vi "Write Version.vi"(8 "error in":errorcluster, 10 "Version":string, 11 "Custom Device Config in":refnum<class "Custom Device Config.lvclass">) -> (0 "error out":errorcluster, 3 "Custom Device Config out":refnum<class "Custom Device Config.lvclass">)   [LabVIEW 2024, in "Parser.lvlib" / "Custom Device Config.lvclass"]
uses:
  Custom Device Config.lvclass
  Custom Device Config.lvclass/Custom Device Config.ctl
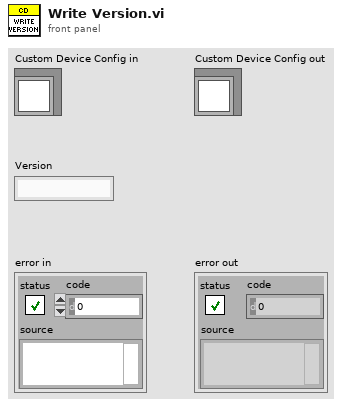
[diagram p1: front panel]
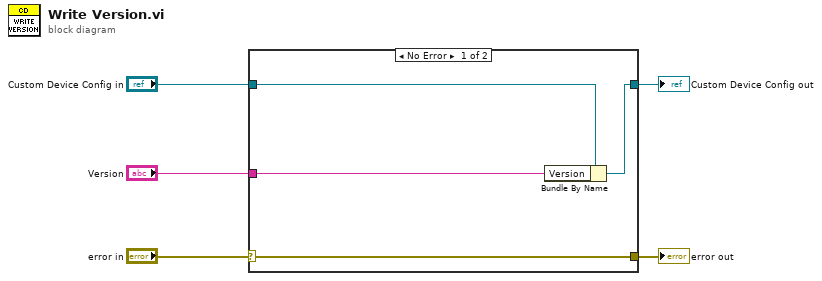
[diagram p0: block diagram]
diagram:
  n1 = case shown="No Error" "error in" {
    selector: "error in" -> [w9 w11]
    tunnel: [w9 w11] -> w4
    tunnel: [w7 w10] -> w2
    tunnel: "Custom Device Config in" -> [w8 w10]
    tunnel: "Version" -> [w6 _]
    frame No Error {
      n2 = Bundle By Name(cluster=w8, "Version"=w6) -> (w7:refnum<class "Custom Device Config.lvclass">)
    }
    frame Error {
    }
  }
  "error out" <- w4
  "Custom Device Config out" <- w2
